vi "Remove padding.vi"(11 "Array in":T2(array[cluster])) -> (3 "Array out":T3[](array[typedef]))   [LabVIEW 2016, in "fgt_SDK.lvlib"]
uses:
  fgt_SDK.lvlib
  TypeDefs/fgt_INSTRUMENT_TYPE.ctl
  TypeDefs/fgt_CHANNEL_INFO.ctl
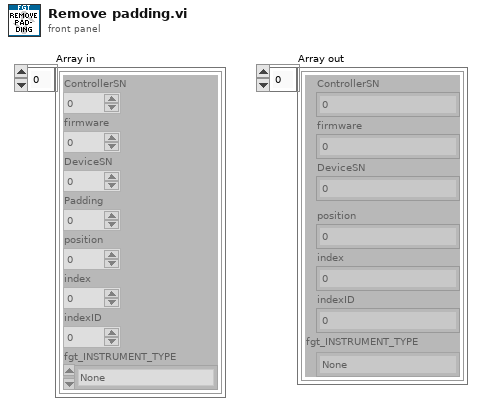
[diagram p1: front panel]
types:
  T1 = typedef "fgt_SDK.lvlib/fgt_INSTRUMENT_TYPE.ctl" = enum32{"None", "MFCS", "MFCS_EZ", "FRP", "LineUP", "IPS"}
  T2 = cluster{"ControllerSN":u16, "firmware":u16, "DeviceSN":u16, "Padding":u16, "position":u32, "index":u32, "indexID":u32, "fgt_INSTRUMENT_TYPE":T1}[]
  T3 = typedef "fgt_SDK.lvlib/fgt_CHANNEL_INFO.ctl" = cluster{"ControllerSN":u16, "firmware":u16, "DeviceSN":u16, "position":u32, "index":u32, "indexID":u32, "fgt_INSTRUMENT_TYPE":T1}
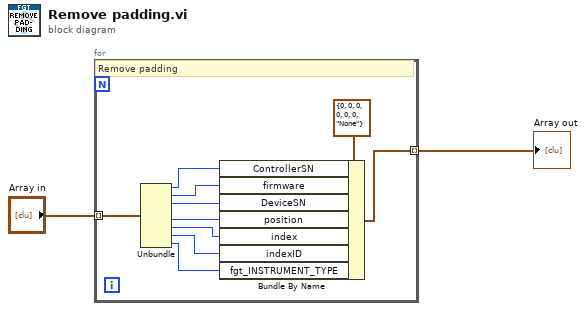
[diagram p0: block diagram]
diagram:
  n1 = for {
    tunnel: "Array in" -> [w12] mode=indexing
    tunnel: [w3] -> w2 mode=indexing
    # "Remove padding"
    n2 = Unbundle(w12) -> ("ControllerSN"=w11:u16, "firmware"=w10:u16, "DeviceSN"=w9:u16, "position"=w8:u32, "index"=w7:u32, "indexID"=w6:u32, "fgt_INSTRUMENT_TYPE"=w5:T1)  [unwired: 1 out]
    n3 = Bundle By Name(cluster=T3 {"ControllerSN"=0, "firmware"=0, "DeviceSN"=0, "position"=0, "index"=0, "indexID"=0, "fgt_INSTRUMENT_TYPE"=enum."None"} ("fgt_CHANNEL_INFO"), "ControllerSN"=w11, "firmware"=w10, "DeviceSN"=w9, "position"=w8, "index"=w7, "indexID"=w6, "fgt_INSTRUMENT_TYPE"=w5) -> (w3:T3)
  }
  "Array out" <- w2
